vi "Instrument Atten Preadjust (LTE).vi"(0 "Session In":refnum<visa-resource-name>="GPIB0::16::INSTR", 1 "ON/OFF":string="ON", 7 "error in":errorcluster {"code" format="%.0x"}, 13 "RO(T)":bool) -> (20 "Session Out":refnum<visa-resource-name>, 26 "Read":string, 27 "error out":errorcluster {"code" format="%.0x"})   [LabVIEW 2018]
doc: "Launches the Instrument I/O Assistant, which you can use to communicate with message-based instruments and graphically parse the response. For example you can communicate with an instrument that uses a serial, Ethernet, or GPIB interface."
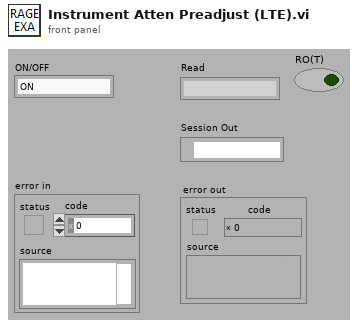
[diagram p1: front panel]
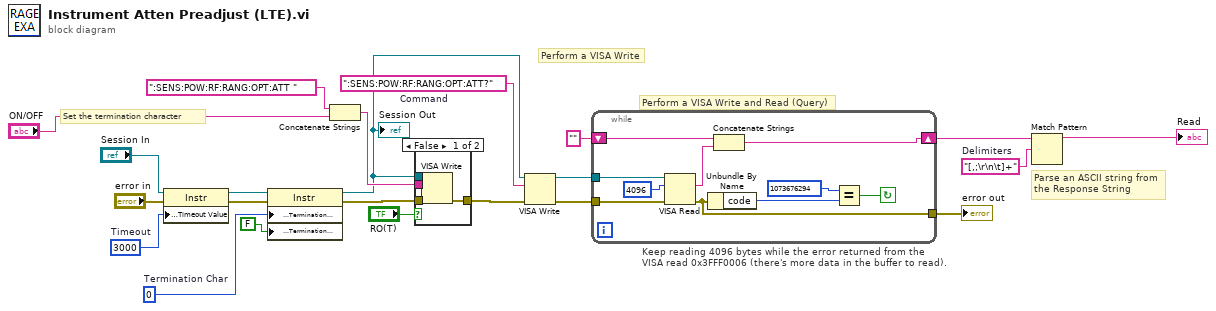
[diagram p0: block diagram]
diagram:
  w4 = "[,;\r\n\t]+"  # Delimiters
  w6 = ":SENS:POW:RF:RANG:OPT:ATT?"  # Command
  w17 = u8 0  # Termination Char
  w21 = u32 3000  # Timeout
  # "Parse an ASCII string from the Response String"
  # "Perform a VISA Write and Read (Query)"
  # "Keep reading 4096 bytes while the error returned from the\nVISA read 0x3FFF0006 (there's more data in the buffer to read)."
  # "Perform a VISA Write"
  # "Set the termination character"
  n1 = property class="Instr"(reference="Session In", error in="error in", "General Settings:Timeout Value"=w21) -> (reference out=w16:refnum<visa-resource-name>, error out=w19:errorcluster)
  n2 = property class="Instr"(reference=w16, error in=w19, "Message Based Settings:Termination Character"=w17, "Message Based Settings:Termination Character Enable"=FALSE ("enable")) -> (reference out=w2:refnum<visa-resource-name>, error out=w18:errorcluster)
  "Session Out" <- w2
  n3 = Concatenate Strings(":SENS:POW:RF:RANG:OPT:ATT " ("staticText"), "ON/OFF") -> (w11:string)
  n4 = case shown="False" "RO(T)" {
    tunnel: w18 -> [w26 w27]
    tunnel: [w25 w27] -> w12
    tunnel: w11 -> [w24 _]
    tunnel: w2 -> [w23 _]
    frame False {
      n5 = VISA Write(VISA resource name=w23, write buffer=w24, error in (no error)=w26) -> (error out=w25:errorcluster)  [unwired: 2 out]
    }
    frame True {
    }
  }
  n6 = VISA Write(VISA resource name=w2, write buffer=w6, error in (no error)=w12) -> (VISA resource name out=w10:refnum<visa-resource-name>, error out=w9:errorcluster)  [unwired: 1 out]
  n7 = while {
    tunnel: w10 -> [w34]
    shift-right: [w28] -> w3
    shift-left: "" -> [w33]
    tunnel: w9 -> [w31]
    tunnel: [w30] -> w8
    stop <- w29 continue-if-true
    n8 = VISA Read(VISA resource name=w34, byte count=u32 4096 ("byte count (0)"), error in (no error)=w31) -> (read buffer=w32:string, error out=w30:errorcluster)  [unwired: 2 out]
    n9 = Unbundle By Name(w30) -> ("code"=w36:i32)
    n10 = Concatenate Strings(w33, w32) -> (w28:string)
    n11 = Equal?(x=1073676294, y=w36) -> (x = y?=w29:bool)
  }
  "error out" <- w8
  n12 = Match Pattern(string=w3, regular expression=w4) -> (before substring=→"Read":string)  [unwired: 4 out]
